vi "start_period_task.vi"(6 "error in":errorcluster, 9 "ClockDL100201DAQmx in":refnum<class "ClockDL100201DAQmx.lvclass">) -> (0 "error out":errorcluster, 3 "GenericClock.lvclass out":refnum<class "ClockDL100201DAQmx.lvclass">)   [LabVIEW 2010, in "ClockDL100201DAQmx.lvclass"]
doc: "This vi configures and starts the period task which will trigger the train task to output a pulse of trains at a given interval."
uses:
  ClockDL100201DAQmx.lvclass
  ClockDL100201DAQmx.lvclass/ClockDL100201DAQmx.ctl
  <vilib>/DAQmx/create/channels.llb/DAQmx Create Channel (CO-Pulse Generation-Frequency).vi
  <vilib>/DAQmx/configure/timing.llb/DAQmx Timing (Implicit).vi
  <vilib>/DAQmx/configure/trigger.llb/DAQmx Start Trigger (Digital Edge).vi
  <vilib>/DAQmx/configure/trigger.llb/DAQmx Start Trigger (None).vi
  Program Files/National Instruments/LabVIEW 2010/resource/objmgr/daqmx.rc
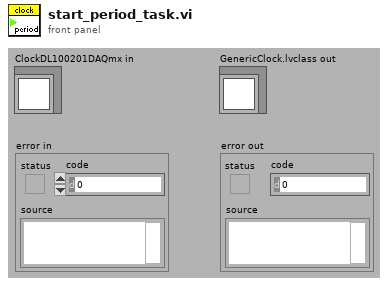
[diagram p1: front panel]
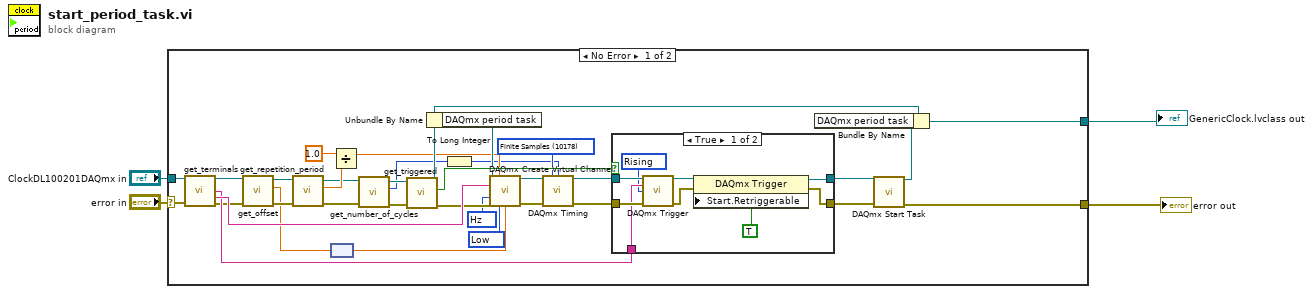
[diagram p0: block diagram]
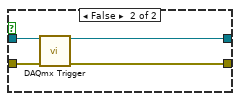
[diagram p2: hidden frame]
diagram:
  n1 = case shown="No Error" "error in" {
    selector: "error in" -> [w12 w54]
    tunnel: "ClockDL100201DAQmx in" -> [w37 w53]
    tunnel: [w14 w53] -> w3
    tunnel: [w13 w54] -> w2
    frame No Error {
      w24 = 10178 items=["Finite Samples"=10178, "Continuous Samples"=10123, "Hardware Timed Single Point"=12522] ("sample mode")
      w22 = 10214 items=["High"=10192, "Low"=10214] ("idle state")
      w21 = 10373 items=["Hz"=10373] ("units")
      n2 = call-dynamic "get_terminals.vi"("ClockDL100201DAQmx in"=w37, "error in (no error)"=w12) -> ("ClockDL100201DAQmx out"=w11:refnum<class "ClockDL100201DAQmx.lvclass">, "trigger source"=w38:tag, "period counter"=w39:tag, "error out"=w10:errorcluster)  [unwired: 9 in, 1 out]
      n3 = call-dynamic "get_offset.vi"("error in (no error)"=w10, "GenericClock.lvclass in"=w11) -> ("error out"=w8:errorcluster, "offset"=w7:dbl[unit], "GenericClock.lvclass out"=w9:refnum<class "ClockDL100201DAQmx.lvclass">)  [unwired: 7 in]
      n4 = call-dynamic "get_repetition_period.vi"("error in (no error)"=w8, "GenericClock.lvclass in"=w9) -> ("error out"=w15:errorcluster, "repetition period"=w17:dbl[unit], "GenericClock.lvclass out"=w16:refnum<class "ClockDL100201DAQmx.lvclass">)  [unwired: 7 in]
      n5 = Divide(x=dbl[unit] 1.0, y=w17) -> (x/y=w19:dbl)
      n6 = node(w7) -> (w6:dbl)
      n7 = call-dynamic "get_number_of_cycles.vi"("error in (no error)"=w15, "GenericClock.lvclass in"=w16) -> ("error out"=w32:errorcluster, "number of cycles"=w25:i64, "GenericClock.lvclass out"=w33:refnum<class "ClockDL100201DAQmx.lvclass">)  [unwired: 7 in]
      n8 = call-dynamic "get_triggered.vi"("error in (no error)"=w32, "GenericClock.lvclass in"=w33) -> ("error out"=w35:errorcluster, "triggered?"=w36:bool, "GenericClock.lvclass out"=w34:refnum<class "ClockDL100201DAQmx.lvclass">)  [unwired: 7 in]
      n9 = Unbundle By Name(w34) -> ("DAQmx period task"=w20:refnum<k21>)
      n10 = To Long Integer(number=w25) -> (32bit integer=w5:i32)
      n11 = call-poly <vilib>:"DAQmx Create Virtual Channel.vi"("task in"=w20, "frequency"=w19, "counter"=w39, "units"=w21, "error in"=w35, "idle state"=w22, "initial delay"=w6) -> ("task out"=w30:refnum<k21>, "error out"=w23:errorcluster)  [unwired: 7 in]
      n12 = call-poly <vilib>:"DAQmx Timing.vi"("task/channels in"=w30, "sample mode"=w24, "samples per channel"=w5, "error in"=w23) -> ("task out"=w26:refnum<k21>, "error out"=w27:errorcluster)  [unwired: 10 in]
      n13 = case shown="True" w36 {
        tunnel: w26 -> [w48 w52]
        tunnel: w27 -> [w47 w51]
        tunnel: [w41 w50] -> w28
        tunnel: [w43 w49] -> w31
        tunnel: w38 -> [w46 _]
        frame True {
          w45 = 10280 items=["Rising"=10280, "Falling"=10171] ("edge")
          n14 = call-poly <vilib>:"DAQmx Trigger.vi"("task/channels in"=w48, "source"=w46, "edge"=w45, "error in"=w47) -> ("task out"=w44:refnum<k21>, "error out"=w42:errorcluster)  [unwired: 10 in]
          n15 = property class="DAQmx Trigger"(reference=w44, error in=w42, "Start.Retriggerable"=TRUE) -> (reference out=w43:refnum<k21>, error out=w41:errorcluster)
        }
        frame False {
          n16 = call-poly <vilib>:"DAQmx Trigger.vi"("task/channels in"=w52, "error in"=w51) -> ("task out"=w49:refnum<k21>, "error out"=w50:errorcluster)  [unwired: 12 in]
        }
      }
      n17 = call <vilib>:"DAQmx Start Task.vi"("task/channels in"=w31, "error in"=w28) -> ("task out"=w29:refnum<k21>, "error out"=w13:errorcluster)  [unwired: 12 in]
      n18 = Bundle By Name(cluster=w34, "DAQmx period task"=w29) -> (w14:refnum<class "ClockDL100201DAQmx.lvclass">)
    }
    frame Error {
    }
  }
  "error out" <- w2
  "GenericClock.lvclass out" <- w3
